vi "projection transformation matching function.vi"(3 "output control":T1, 4 "data":variant, 5 "X":dbl[](array[numeric])) -> (0 "error out":errorcluster, 1 "gradient":dbl[](array[numeric]), 2 "f(X)":dbl)   [LabVIEW 2024]
doc: "Use this template VI as a starting point to create an objective function you want to pass to the Unconstrained Optimization VI."
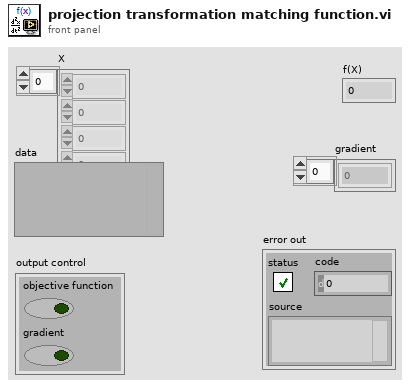
[diagram p1: front panel]
types:
  T1 = cluster{"objective function":bool, "gradient":bool}
  T2 = cluster{"Interpolation Type":enum32{"Zero Order", "Bilinear", "Quadratic", "Cubic", "Bilinear Fixed"}, "Destination Width":u32, "Destination Height":u32, "Fill Value":sgl}
  T3 = cluster{"template":u8[][], "target img":u8[][], "image size":dbl[]}
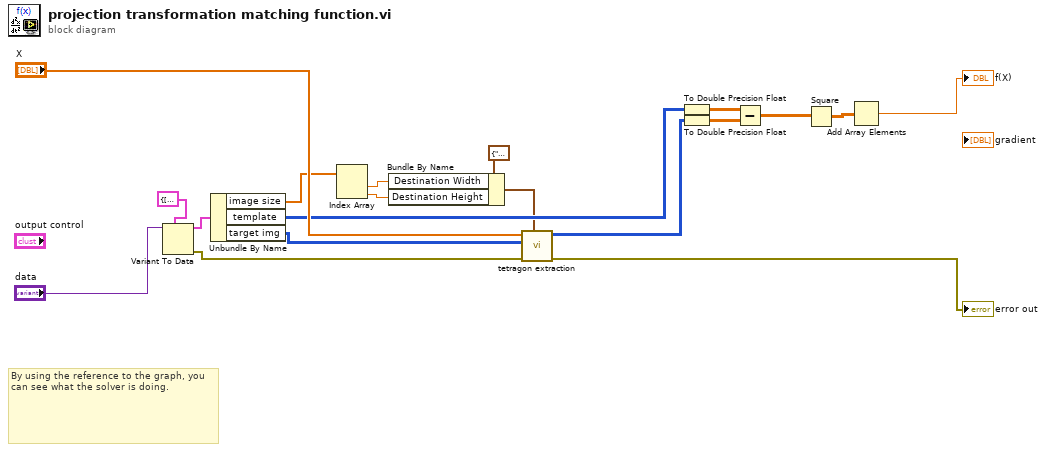
[diagram p0: block diagram]
diagram:
  # "By using the reference to the graph, you can see what the solver is doing."
  n1 = Variant To Data(type=T3 {"template"=[], "target img"=[], "image size"=[]}, Variant="data") -> (data=w15:T3, error out=w10:errorcluster)  [unwired: 1 in]
  n2 = Unbundle By Name(w15) -> ("image size"=w4:dbl[], "template"=w12:u8[][], "target img"=w13:u8[][])
  n3 = Index Array(array=w4) -> (element #1=w3:dbl, element #2=w2:dbl)  [unwired: 2 in]
  n4 = Bundle By Name(cluster=T2 {"Interpolation Type"=enum."Bilinear", "Destination Width"=0, "Destination Height"=0, "Fill Value"=0.0} ("Options"), "Destination Width"=w3, "Destination Height"=w2) -> (w1:T2)
  n5 = call "tetragon extraction.vi"("Options"=w1, "error in (no error)"=w10, "target img"=w13, "X"="X") -> ("error out"=→"error out":errorcluster, "Image Pixels (U8)"=w11:u8[][])  [unwired: 5 in, 1 out]
  n6 = To Double Precision Float(number=w12) -> (double precision float=w8:dbl[][])
  n7 = To Double Precision Float(number=w11) -> (double precision float=w7:dbl[][])
  n8 = Subtract(x=w8, y=w7) -> (x-y=w19:dbl[][])
  n9 = Square(x=w19) -> (x^2=w18:dbl[][])
  n10 = Add Array Elements(numeric array=w18) -> (sum=→"f(X)":dbl)
